vi "Fit.vi"(8 "error in (no error)":errorcluster caption="entrée d'erreur (pas d'erreur)", 9 "y":string[][](array[string]), 10 "X":string[][](array[string]), 11 "AdditiveChi2Sampler.lvclass":refnum<class "AdditiveChi2Sampler.lvclass">) -> (0 "error out":errorcluster caption="sortie d'erreur", 2 "String Data":string, 3 "AdditiveChi2Sampler.lvclass":refnum<class "AdditiveChi2Sampler.lvclass">)   [LabVIEW 2020, in "AdditiveChi2Sampler.lvclass"]
doc: "Set the parameters\n\nReturns : \n\n- String : OK"
uses:
  AdditiveChi2Sampler.lvclass
  AdditiveChi2Sampler.lvclass/AdditiveChi2Sampler.ctl
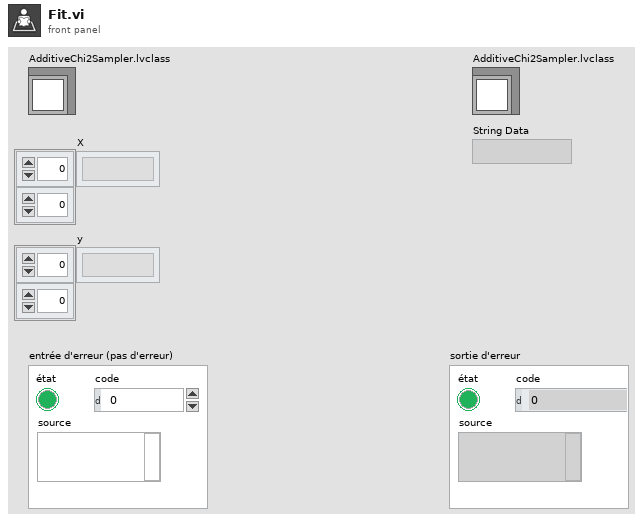
[diagram p1: front panel]
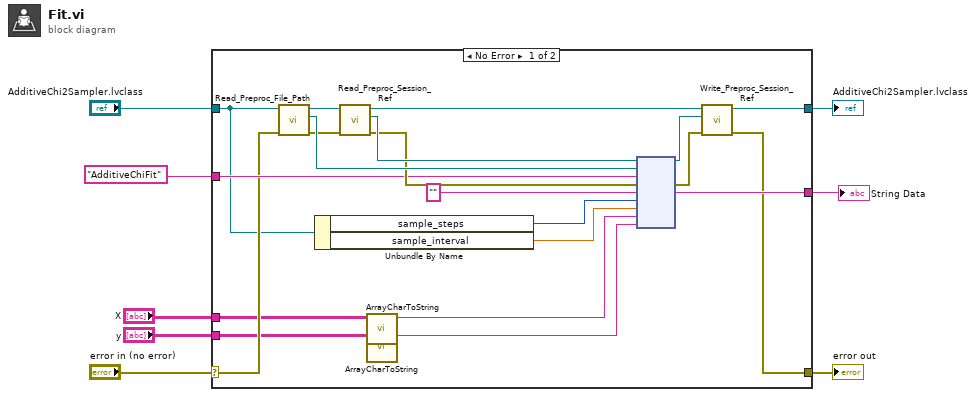
[diagram p0: block diagram]
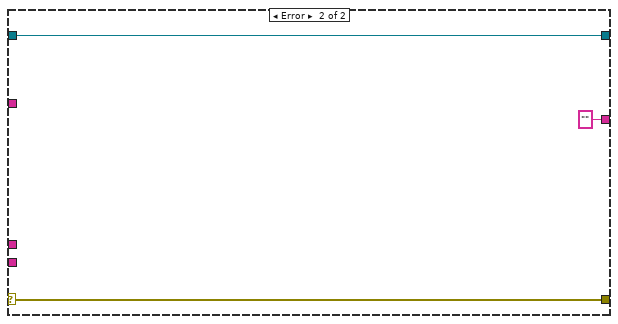
[diagram p2: hidden frame]
diagram:
  n1 = case shown="No Error" "error in (no error)" {
    selector: "error in (no error)" -> [w17 w32]
    tunnel: [w13 w32] -> w7
    tunnel: [w15 w31] -> w5
    tunnel: "AdditiveChi2Sampler.lvclass" -> [w14 w31]
    tunnel: "AdditiveChiFit" ("Fonction") -> [w18 _]
    tunnel: "X" -> [w12 _]
    tunnel: [w16 ""] -> w2
    tunnel: "y" -> [w10 _]
    frame No Error {
      n2 = call-dynamic "Read_Preproc_File_Path.vi"("error in (no error)"=w17, "Python in"=w14) -> ("error out"=w24:errorcluster, "File_Path"=w27:path, "Python out"=w29:refnum<class "AdditiveChi2Sampler.lvclass">)  [unwired: 7 in]
      n3 = Unbundle By Name(w14) -> ("sample_steps"=w20:i32, "sample_interval"=w19:dbl)
      n4 = call-dynamic "Read_Preproc_Session_Ref.vi"("error in (no error)"=w24, "Python in"=w29) -> ("error out"=w25:errorcluster, "Session_ref"=w26:refnum<k35>, "Python out"=w28:refnum<class "AdditiveChi2Sampler.lvclass">)  [unwired: 7 in]
      n5 = call "ArrayCharToString.vi"("TAB"=w12) -> ("Instruction"=w11:string)  [unwired: 10 in]
      n6 = call "ArrayCharToString.vi"("TAB"=w10) -> ("Instruction"=w9:string)  [unwired: 10 in]
      n7 = node(w26, w27, w18, w25, "", w20, w19, w11, w9) -> (w21:refnum<k35>, w23:errorcluster, w16:string)  [unwired: 4 in, 2 out]
      n8 = call-dynamic "Write_Preproc_Session_Ref.vi"("error in (no error)"=w23, "Session_ref"=w21, "Python in"=w28) -> ("error out"=w13:errorcluster, "Python out"=w15:refnum<class "AdditiveChi2Sampler.lvclass">)  [unwired: 7 in]
    }
    frame Error {
    }
  }
  "error out" <- w7
  "AdditiveChi2Sampler.lvclass" <- w5
  "String Data" <- w2
